vi "例4-35.vi"() -> ()   [LabVIEW 2019]
uses:
  <vilib>/Native 3D Graph/xcontrol/3DPC_SurfacePlot.xctl
panel:
  out "3D Graph":refnum<class "Base Datatype.lvclass">[](xcontrol) caption="三维图形"
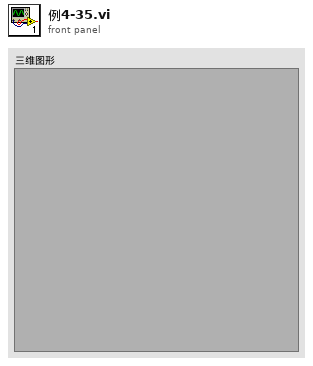
[diagram p1: front panel]
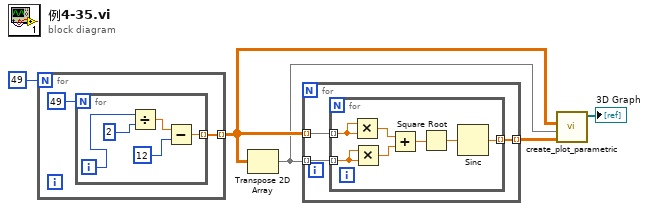
[diagram p0: block diagram]
diagram:
  n1 = for {
    N: 49 -> [_]
    tunnel: [w6] -> w2 mode=indexing
    n2 = for {
      N: 49 -> [_]
      tunnel: [w8] -> w6 mode=indexing
      i -> [w10]
      n3 = Divide(x=w10, y=2) -> (x/y=w12:dbl)
      n4 = Subtract(x=w12, y=12) -> (x-y=w8:dbl)
    }
  }
  n5 = Transpose 2D Array(2D array=w2) -> (transposed array=w1:dbl[][])
  n6 = for {
    tunnel: w2 -> [w15] mode=indexing
    tunnel: w1 -> [w14] mode=indexing
    tunnel: [w13] -> w3 mode=indexing
    n7 = for {
      tunnel: w15 -> [w19] mode=indexing
      tunnel: w14 -> [w18] mode=indexing
      tunnel: [w16] -> w13 mode=indexing
      n8 = Multiply(x=w19, y=w19) -> (x*y=w22:dbl)
      n9 = Multiply(x=w18, y=w18) -> (x*y=w17:dbl)
      n10 = Add(x=w22, y=w17) -> (x+y=w21:dbl)
      n11 = Square Root(x=w21) -> (sqrt(x)=w20:dbl)
      n12 = Sinc(1:w20) -> (0:w16:dbl)
    }
  }
  n13 = call <vilib>:"create_plot_parametric.vi"("z matrix"=w3, "y matrix"=w1, "x matrix"=w2) -> ("plots out"=→"3D Graph":refnum<class "Base Datatype.lvclass">[])  [unwired: 2 in, 6 out]
